vi "CloseRG.vi"(2 "error out":errorcluster, 3 "VISA resource name out":refnum<visa-resource-name>) -> (0 "return count 3":u32, 1 "return count 4":u32)   [LabVIEW 2009]
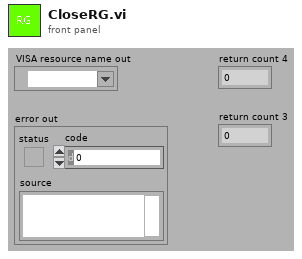
[diagram p1: front panel]
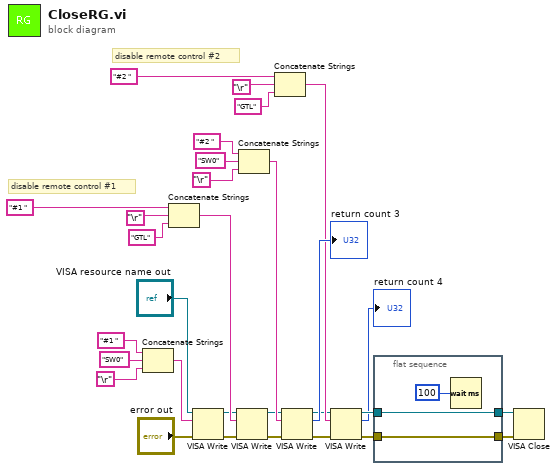
[diagram p0: block diagram]
diagram:
  # "disable remote control #1"
  # "disable remote control #2"
  n1 = Concatenate Strings("#1 " ("format string"), "SW0" ("initial string"), "\r" ("input 1")) -> (w14:string)
  n2 = Concatenate Strings("#1 " ("initial string"), "\r", "GTL" ("input 1")) -> (w7:string)
  n3 = VISA Write(VISA resource name="VISA resource name out", write buffer=w14, error in (no error)="error out") -> (VISA resource name out=w2:refnum<visa-resource-name>, error out=w5:errorcluster)  [unwired: 1 out]
  n4 = VISA Write(VISA resource name=w2, write buffer=w7, error in (no error)=w5) -> (VISA resource name out=w1:refnum<visa-resource-name>, error out=w4:errorcluster)  [unwired: 1 out]
  n5 = Concatenate Strings("#2 " ("format string"), "SW0" ("initial string"), "\r" ("input 1")) -> (w24:string)
  n6 = Concatenate Strings("#2 " ("initial string"), "\r", "GTL" ("input 1")) -> (w23:string)
  n7 = VISA Write(VISA resource name=w1, write buffer=w24, error in (no error)=w4) -> (VISA resource name out=w21:refnum<visa-resource-name>, return count=→"return count 3":u32, error out=w22:errorcluster)
  n8 = VISA Write(VISA resource name=w21, write buffer=w23, error in (no error)=w22) -> (VISA resource name out=w28:refnum<visa-resource-name>, return count=→"return count 4":u32, error out=w27:errorcluster)
  n9 = flat-sequence {
    tunnel: w28 -> [w32]
    tunnel: w27 -> [w31]
    tunnel: [w32] -> w29
    tunnel: [w31] -> w30
    frame #0 {
      n10 = Wait (ms)(milliseconds to wait=u32 100) -> ()  [unwired: 1 out]
    }
  }
  n11 = VISA Close(VISA resource name=w29, error in (no error)=w30) -> ()  [unwired: 1 out]
